vi "Initialize Data Channels.vi"(8 "error in (no error)":errorcluster, 11 "6952A in":refnum<class "69X_79X.lvclass">) -> (0 "error out":errorcluster, 3 "6952A out":refnum<class "69X_79X.lvclass">)   [LabVIEW 2019]
uses:
  69X_79X.lvclass
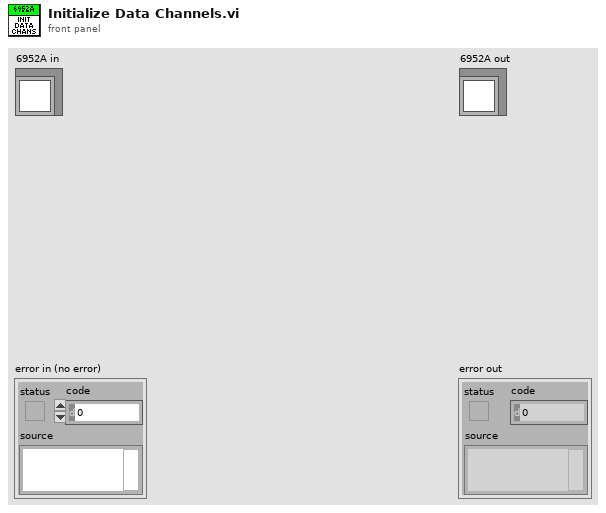
[diagram p1: front panel]
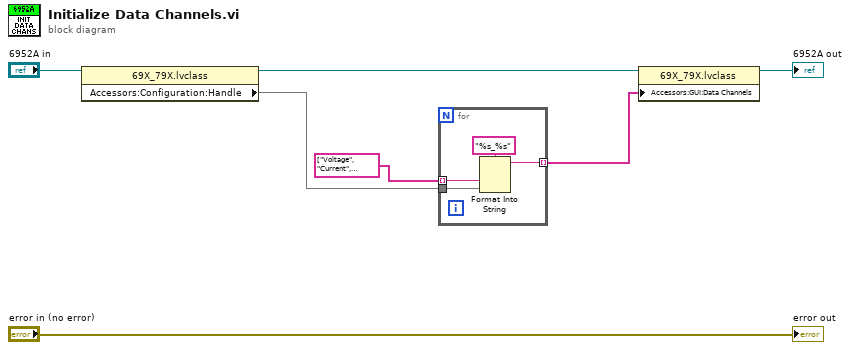
[diagram p0: block diagram]
diagram:
  n1 = property class="69X_79X.lvclass"(reference="6952A in") -> (reference out=w1:refnum<class "69X_79X.lvclass">, "Accessors:Configuration:Handle"=w7)  [unwired: 1 in, 1 out]
  n2 = for {
    tunnel: w7 -> [w10]
    tunnel: string[] ["Voltage", "Current", "Output", "Interlock", "OCP", "OVP"] -> [w9] mode=indexing
    tunnel: [w8] -> w6 mode=indexing
    n3 = Format Into String(format string="%s_%s", w9, w10) -> (resulting string=w8:string)  [unwired: 2 in, 1 out]
  }
  n4 = property class="69X_79X.lvclass"(reference=w1, "Accessors:GUI:Data Channels"=w6) -> (reference out=→"6952A out":refnum<class "69X_79X.lvclass">)  [unwired: 1 in, 1 out]
  "error out" <- "error in (no error)"
